vi "RPC Method veristand Read.vi"(8 "error in (no error)":errorcluster, 11 "OOP Server in":refnum<class "veristand-grpc.lvclass">) -> (0 "error out":errorcluster, 3 "OOP Server out":refnum<class "veristand-grpc.lvclass">)   [LabVIEW 2021, in "Veristandgrpc_server.lvlib" / "veristand-grpc.lvclass"]
uses:
  veristand-grpc.lvclass
  veristand-grpc.lvclass/veristand-grpc.ctl
  Data/Data Server.lvclass/Data Server.ctl
  Data/Read.vi
  RPC Messages/Get veristand_Request.vi
  RPC Messages/Set veristand_Reponse.vi
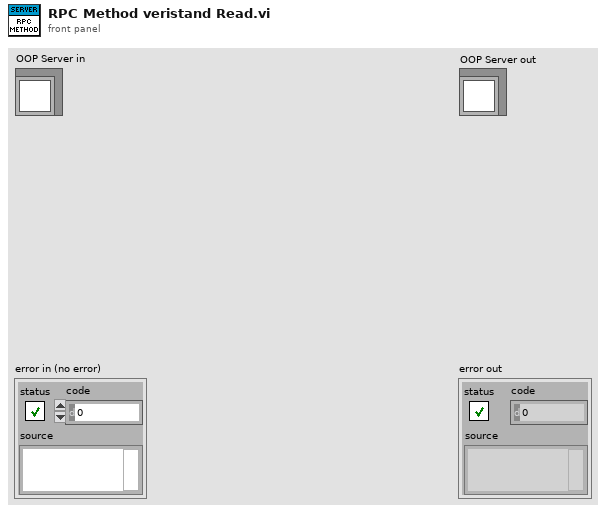
[diagram p1: front panel]
types:
  T1 = typedef "Veristandgrpc_server.lvlib/veristand-grpc.lvclass/Server Internal UEs.ctl" = cluster{"veristand Write Internal UE":refnum<user-event>, "veristand Read Internal UE":refnum<user-event>}
  T2 = typedef "Veristandgrpc_server.lvlib/veristand-grpc.lvclass/Server gRPC UEs.ctl" = cluster{"veristand Write gRPC UE":refnum<user-event>, "veristand Read gRPC UE":refnum<user-event>}
  T3 = typedef "grpc-lvsupport-release.lvlib/grpcId.ctl" = u64
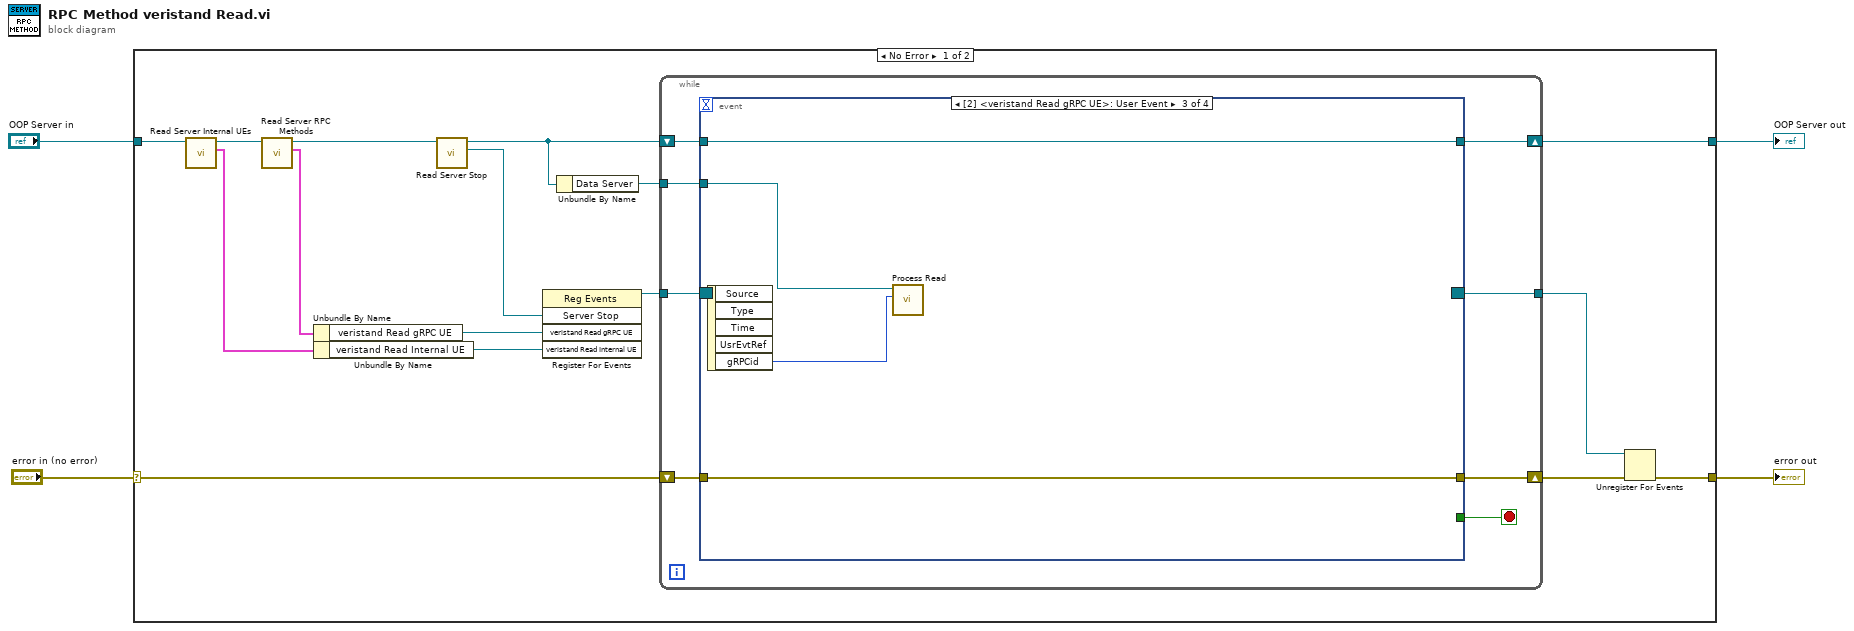
[diagram p0: block diagram]
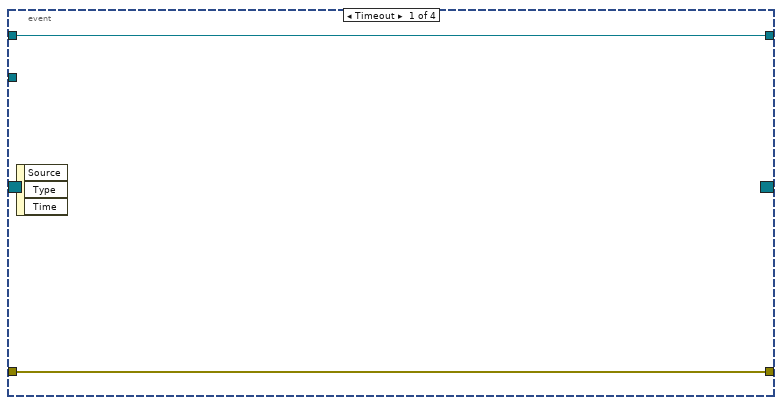
[diagram p2: hidden frame]
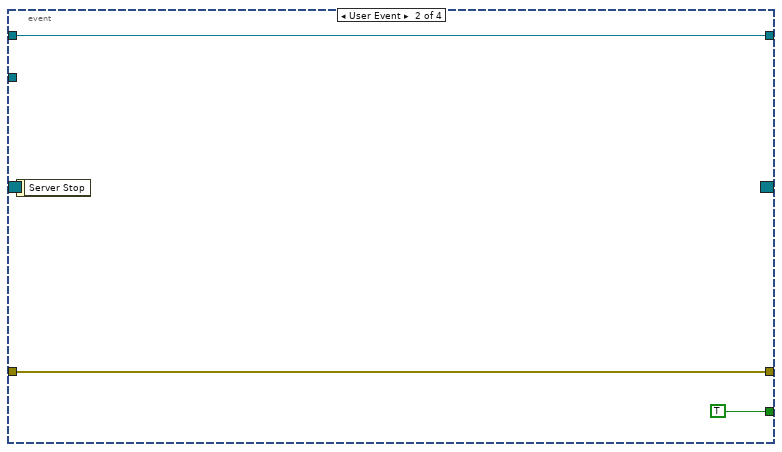
[diagram p3: hidden frame]
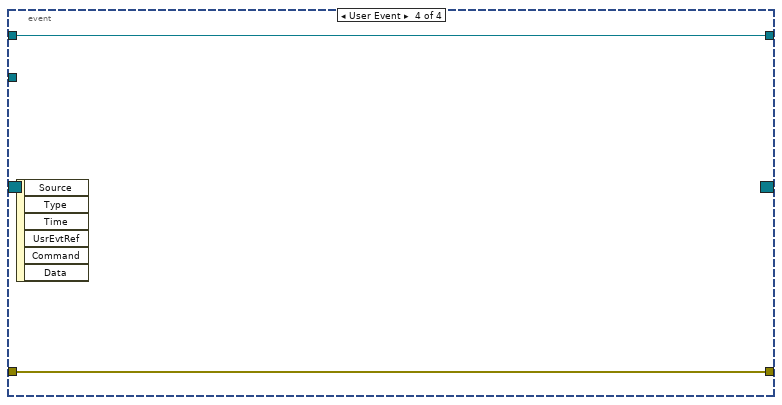
[diagram p4: hidden frame]
diagram:
  n1 = case shown="No Error" "error in (no error)" {
    selector: "error in (no error)" -> [w16 w41]
    tunnel: [w14 w41] -> w3
    tunnel: "OOP Server in" -> [w18 w40]
    tunnel: [w7 w40] -> w1
    frame No Error {
      n2 = call "Read Server Internal UEs.vi"("SignalGeneratorService in"=w18) -> ("Server Internal UEs"=w10:T1, "SignalGeneratorService out"=w17:refnum<class "veristand-grpc.lvclass">)  [unwired: 8 in, 1 out]
      n3 = call "Read Server RPC Methods.vi"("SignalGeneratorService in"=w17) -> ("Server RPC Methods"=w12:T2, "SignalGeneratorService out"=w8:refnum<class "veristand-grpc.lvclass">)  [unwired: 8 in, 1 out]
      n4 = Unbundle By Name ("Unbundle gRPC UE")(w12) -> ("veristand Read gRPC UE"=w11:refnum<user-event>)
      n5 = Unbundle By Name ("Unbundle Internal UE")(w10) -> ("veristand Read Internal UE"=w9:refnum<user-event>)
      n6 = call-dynamic "Read Server Stop.vi"("iService in"=w8) -> ("Server Stop"=w20:refnum<user-event>, "iService out"=w6:refnum<class "veristand-grpc.lvclass">)  [unwired: 8 in, 1 out]
      n7 = register-events(w20, w11, w9) -> (reference out=w19:refnum<event-registration>)  [unwired: 2 in, 1 out]
      n8 = Unbundle By Name(w6) -> ("Data Server"=w5:refnum<class "Data Server.lvclass">)
      n9 = while {
        tunnel: w19 -> [w28]
        tunnel: [w24] -> w13
        shift-right: [w25] -> w15
        shift-left: w16 -> [w26]
        shift-right: [w22] -> w7
        shift-left: w6 -> [w23]
        tunnel: w5 -> [w21]
        stop <- w27 stop-if-true
        n10 = event "RPC Method Event Structure" shown="[2] <veristand Read gRPC UE>: User Event" {
          selector: w28 -> [_ _ _ _]
          dyn-events: [_ _ _ _] -> w24
          timeout: _ -> [_ _ _ _]
          tunnel: [_ TRUE _ _] -> w27
          tunnel: w26 -> [w30 w32 w37 w39]
          tunnel: [w30 w32 w37 w39] -> w25
          tunnel: w23 -> [w29 w31 w36 w38]
          tunnel: [w29 w31 w36 w38] -> w22
          tunnel: w21 -> [_ _ w35 _]
          event Timeout {
            n11 = event-data() -> ()  [unwired: 1 in, 3 out]
          }
          event User Event {
            n12 = event-data() -> ()  [unwired: 1 in, 1 out]
          }
          event User Event {
            n13 = event-data() -> ("gRPCid"=w34:T3)  [unwired: 1 in, 4 out]
            n14 = call "Process Read.vi"("gRPCid"=w34, "Data Server"=w35) -> ()  [unwired: 9 in, 1 out]
          }
          event User Event {
            n15 = event-data() -> ()  [unwired: 1 in, 6 out]
          }
        }
      }
      n16 = Unregister For Events(event registration refnum=w13, error in=w15) -> (error out=w14:errorcluster)
    }
    frame Error {
    }
  }
  "error out" <- w3
  "OOP Server out" <- w1
